vi "Execution Module - GCODE.vi"(5 "Axis Resources":refnum<k21>[](array[refnum])=["Axis 1", "Axis 2", "Axis 3", "Axis 4", "Axis 5"], 7 "Coordinate Space Resource":refnum<k21>="Coordinate Space 1", 8 "error in (no error)":errorcluster, 9 "GCode CMD":T3, 10 "Motion Parameters":T1={"timeout"=-1.0, "acceleration"=1000000000.0, "deceleration"=1000000000.0, "accel. jerk"=1000000.0, "decel. jerk"=1000000.0, "blend mode"=10551334, "blend delay"=-1.0, "smoothing"=0.5, "last blend"=FALSE} {"blend mode" items=["At Profile Complete"=10551335, "At Deceleration"=10551334, "After Delay"=10551336]}) -> (0 "error out":errorcluster, 1 "Speed Request":dbl, 2 "Motion Parameters Out":T1={"timeout"=-1.0, "acceleration"=1000000000.0, "deceleration"=1000000000.0, "accel. jerk"=1000000.0, "decel. jerk"=1000000.0, "blend mode"=10551334, "blend delay"=-1.0, "smoothing"=0.5, "last blend"=FALSE} {"blend mode" items=["At Profile Complete"=10551335, "At Deceleration"=10551334, "After Delay"=10551336]})   [LabVIEW 2014]
uses:
  GCode Parser/GCode Command Cluster.ctl
  Typedefs/Motion Parameters.ctl
  <vilib>/Motion/Express/_s/nimc.fb.straightLineMove.blendMode.ctl
  <vilib>/Motion/Express/_s/nimc.ex.straightLineMove.startStraightLineMove.coordinate.modeAbsolute.blendEnable.1.vi
  <vilib>/Motion/Express/_s/nimc.ex.arcMove.startArcMove.coordinate.modeCircular.blendEnable.1.vi
  <vilib>/Motion/Express/_s/nimc.ex.resetPosition.resetPosition.axis.vi
  <vilib>/Motion/BlockNode/FB.NIMotion.xnode
  <vilib>/Motion/Express/_s/nimc.fb.arcMove.blendMode.ctl
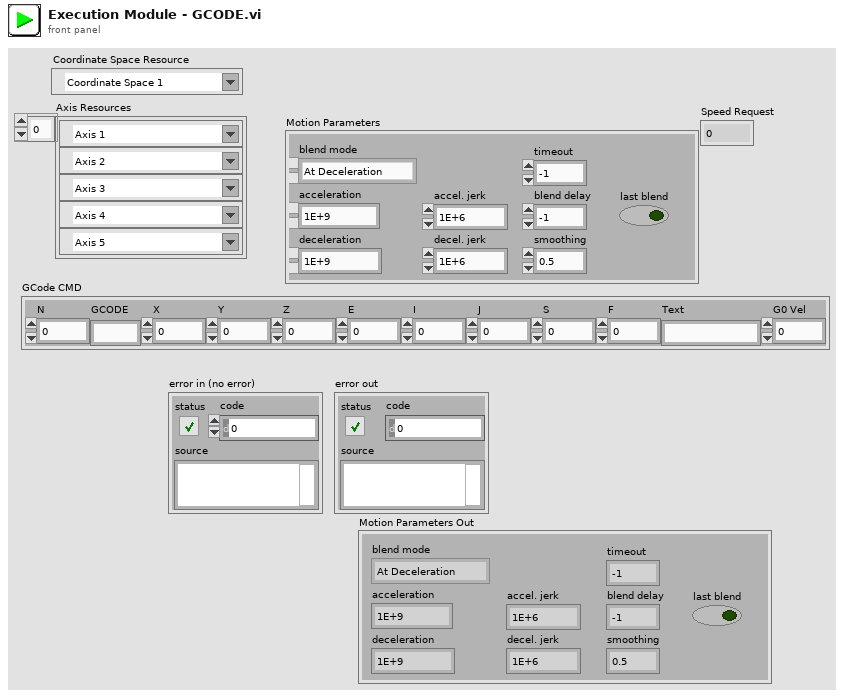
[diagram p1: front panel]
types:
  T1 = typedef "Motion Parameters.ctl" = cluster{"timeout":dbl, "acceleration":dbl, "deceleration":dbl, "accel. jerk":dbl, "decel. jerk":dbl, "blend mode":T2, "blend delay":dbl, "smoothing":dbl, "last blend":bool}
  T2 = typedef "nimc.fb.straightLineMove.blendMode.ctl" = i32
  T3 = typedef "GCode Command Cluster.ctl" = cluster{"N":dbl, "GCODE":string, "X":dbl, "Y":dbl, "Z":dbl, "E":dbl, "I":dbl, "J":dbl, "S":dbl, "F":dbl, "Text":string, "G0 Vel":dbl}
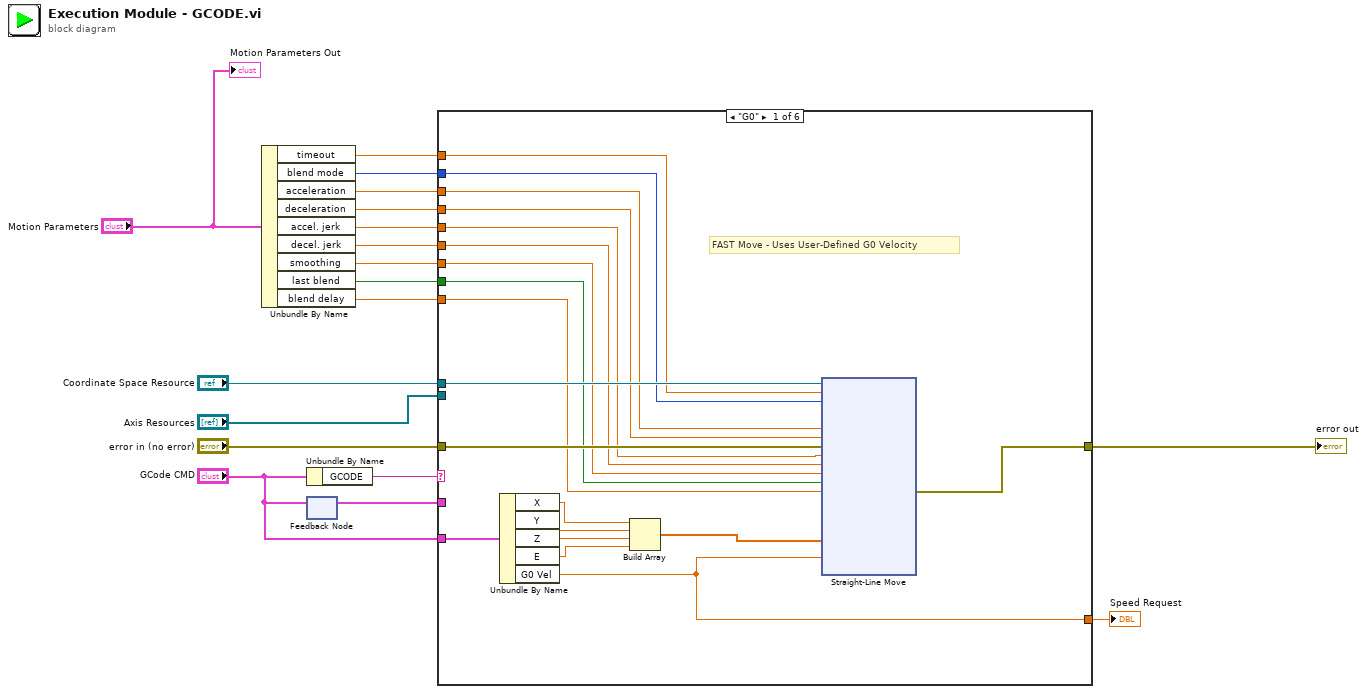
[diagram p0: block diagram]
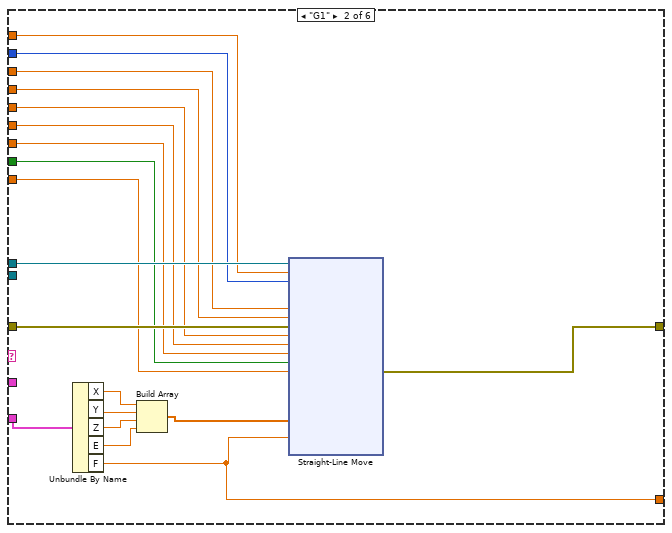
[diagram p2: hidden frame]
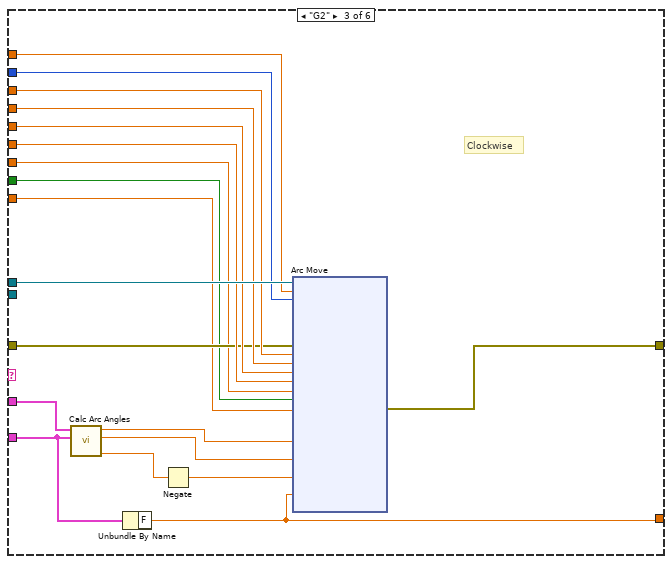
[diagram p3: hidden frame]
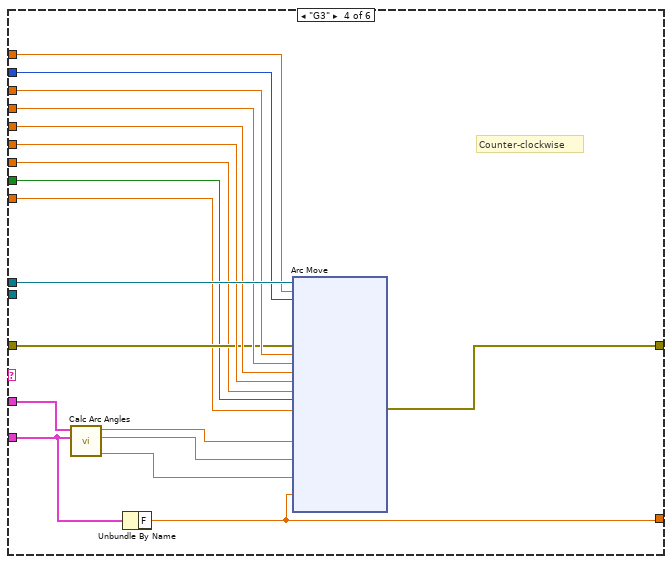
[diagram p4: hidden frame]
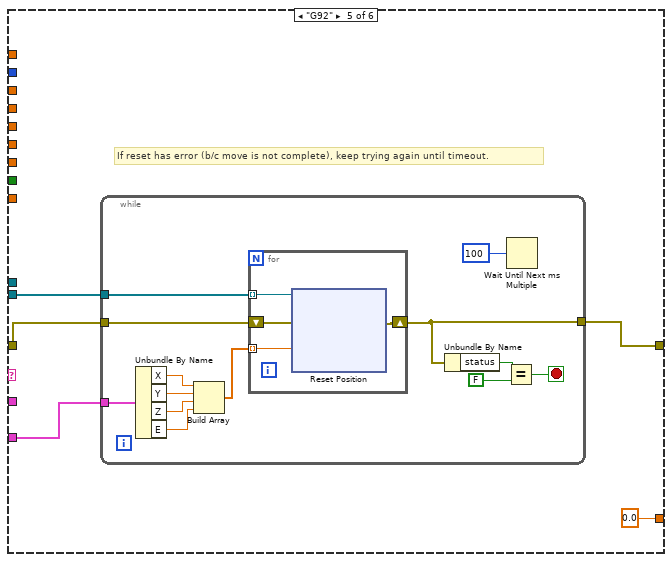
[diagram p5: hidden frame]
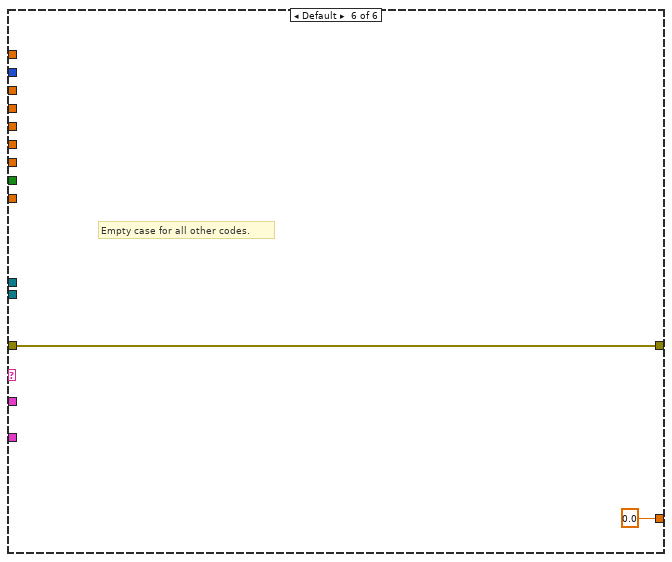
[diagram p6: hidden frame]
diagram:
  n1 = Unbundle By Name("Motion Parameters") -> ("timeout"=w8:dbl, "blend mode"=w9:T2, "acceleration"=w10:dbl, "deceleration"=w11:dbl, "accel. jerk"=w12:dbl, "decel. jerk"=w13:dbl, "smoothing"=w15:dbl, "last blend"=w14:bool, "blend delay"=w16:dbl)
  n2 = Unbundle By Name("GCode CMD") -> ("GCODE"=w3:string)
  n3 = feedback #1() -> (w18:T3)  [unwired: 1 in]
  n4 = feedback-in #1("GCode CMD") -> ()
  n5 = case shown="\"G0\"" w3 {
    tunnel: "Coordinate Space Resource" -> [w31 w69 w115 w155 _ _]
    tunnel: [w37 w76 w105 w145 w179 w206] -> w4
    tunnel: "GCode CMD" -> [w32 w71 w112 w152 w180 _]
    tunnel: "error in (no error)" -> [w30 w68 w106 w146 w181 w206]
    tunnel: w8 -> [w29 w67 w111 w151 _ _]
    tunnel: w9 -> [w28 w66 w98 w140 _ _]
    tunnel: w10 -> [w23 w65 w110 w150 _ _]
    tunnel: w11 -> [w22 w64 w109 w149 _ _]
    tunnel: w12 -> [w21 w63 w108 w148 _ _]
    tunnel: w13 -> [w20 w62 w107 w147 _ _]
    tunnel: w15 -> [w27 w61 w99 w141 _ _]
    tunnel: w14 -> [w26 w60 w100 w142 _ _]
    tunnel: w16 -> [w25 w59 w101 w143 _ _]
    tunnel: "Axis Resources" -> [_ _ _ _ w182 _]
    tunnel: w18 -> [_ _ w114 w154 _ _]
    tunnel: [w19 w58 w97 w138 0.0 ("F") 0.0 ("F")] -> w1
    frame "G0" {
      # "FAST Move - Uses User-Defined G0 Velocity"
      n6 = Unbundle By Name(w32) -> ("X"=w36:dbl, "Y"=w35:dbl, "Z"=w34:dbl, "E"=w33:dbl, "G0 Vel"=w19:dbl)
      n7 = Build Array(w36, w35, w34, w33) -> (w24:dbl[])
      n8 = xnode ("Straight-Line Move")("position[]"=w24, "velocity"=w19, "resource"=w31, "timeout"=w29, "blend mode"=w28, "acceleration"=w23, "deceleration"=w22, "error in"=w30, "accel. jerk"=w21, "decel. jerk"=w20, "smoothing"=w27, "last blend"=w26, "blend delay"=w25) -> ("error out"=w37:errorcluster)  [unwired: 2 out]
    }
    frame "G1" {
      n9 = Unbundle By Name(w71) -> ("X"=w75:dbl, "Y"=w74:dbl, "Z"=w73:dbl, "E"=w72:dbl, "F"=w58:dbl)
      n10 = Build Array(w75, w74, w73, w72) -> (w70:dbl[])
      n11 = xnode ("Straight-Line Move")("position[]"=w70, "velocity"=w58, "resource"=w69, "timeout"=w67, "blend mode"=w66, "acceleration"=w65, "deceleration"=w64, "error in"=w68, "accel. jerk"=w63, "decel. jerk"=w62, "smoothing"=w61, "last blend"=w60, "blend delay"=w59) -> ("error out"=w76:errorcluster)  [unwired: 2 out]
    }
    frame "G2" {
      # "Clockwise"
      n12 = call "Calc Arc Angles.vi"("Arc CMD"=w112, "Initial CMD"=w114) -> ("travel angle out"=w103:dbl, "start angle (tangent)"=w102:dbl, "R"=w113:dbl)  [unwired: 7 in]
      n13 = Unbundle By Name(w112) -> ("F"=w97:dbl)
      n14 = Negate(x=w103) -> (-x=w104:dbl)
      n15 = xnode ("Arc Move")("radius"=w113, "start angle"=w102, "travel angle"=w104, "velocity"=w97, "resource"=w115, "timeout"=w111, "blend mode"=w98, "error in"=w106, "acceleration"=w110, "deceleration"=w109, "accel. jerk"=w108, "decel. jerk"=w107, "smoothing"=w99, "last blend"=w100, "blend delay"=w101) -> ("error out"=w105:errorcluster)  [unwired: 2 out]
    }
    frame "G3" {
      # "Counter-clockwise"
      n16 = call "Calc Arc Angles.vi"("Arc CMD"=w152, "Initial CMD"=w154) -> ("travel angle out"=w139:dbl, "start angle (tangent)"=w144:dbl, "R"=w153:dbl)  [unwired: 7 in]
      n17 = Unbundle By Name(w152) -> ("F"=w138:dbl)
      n18 = xnode ("Arc Move")("radius"=w153, "start angle"=w144, "travel angle"=w139, "velocity"=w138, "resource"=w155, "timeout"=w151, "blend mode"=w140, "error in"=w146, "acceleration"=w150, "deceleration"=w149, "accel. jerk"=w148, "decel. jerk"=w147, "smoothing"=w141, "last blend"=w142, "blend delay"=w143) -> ("error out"=w145:errorcluster)  [unwired: 2 out]
    }
    frame "G92" {
      # "If reset has error (b/c move is not complete), keep trying again until timeout."
      n19 = while {
        tunnel: [w192] -> w179
        tunnel: w182 -> [w190]
        tunnel: w181 -> [w189]
        tunnel: w180 -> [w184]
        stop <- w191 stop-if-true
        n20 = Unbundle By Name(w184) -> ("X"=w188:dbl, "Y"=w187:dbl, "Z"=w186:dbl, "E"=w185:dbl)
        n21 = Build Array(w188, w187, w186, w185) -> (w183:dbl[])
        n22 = for {
          tunnel: w190 -> [w198] mode=indexing
          shift-right: [w199] -> w192
          shift-left: w189 -> [w197]
          tunnel: w183 -> [w196] mode=indexing
          n23 = xnode ("Reset Position")("position"=w196, "resource"=w198, "error in"=w197) -> ("error out"=w199:errorcluster)  [unwired: 1 out]
        }
        n24 = Unbundle By Name(w192) -> ("status"=w194:bool)
        n25 = Equal?(x=w194, y=FALSE) -> (x = y?=w191:bool)
        n26 = Wait Until Next ms Multiple(millisecond multiple=u32 100) -> ()  [unwired: 1 out]
      }
    }
    frame Default {
      # "Empty case for all other codes."
    }
  }
  "error out" <- w4
  "Speed Request" <- w1
  "Motion Parameters Out" <- "Motion Parameters"
